vi "DMMP_GetSamplingInterval.vi"(3 "Input DMMP":refnum<class "DMMP.lvclass">) -> (0 "Sampling Interval (ms)":dbl, 1 "Output DMMP":refnum<class "DMMP.lvclass">)   [LabVIEW 2014, in "DMMP.lvclass"]
uses:
  DMMP.lvclass
  DMMP.lvclass/DMMP.ctl
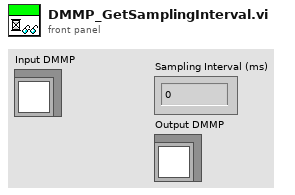
[diagram p1: front panel]
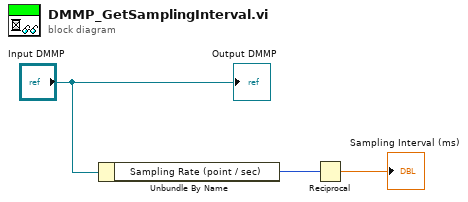
[diagram p0: block diagram]
diagram:
  n1 = Unbundle By Name("Input DMMP") -> ("Sampling Rate (point / sec)"=w2:u32)
  n2 = Reciprocal(x=w2) -> (1/x=→"Sampling Interval (ms)":dbl)
  "Output DMMP" <- "Input DMMP"
